vi "PH_PILS.Action _Cerpass.vi"(0 "i ref in":refnum<vi>, 2 "Service Name":string="N/A", 5 "error in":errorcluster) -> (14 "i ref out":refnum<vi>, 19 "error out":errorcluster)   [LabVIEW 2014, in "PH_PILS.lvlib"]
doc: "This VI sets the Cerpass GUI element."
uses:
  PH_PILS.lvlib
  PH_PILS.Operation Mode.ctl
  PH_Basics/PH_Common/PH_Common.lvlib
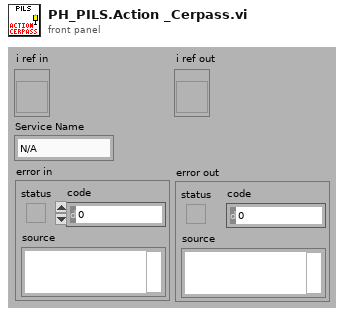
[diagram p1: front panel]
types:
  T1 = typedef "PH_PILS.lvlib/PH_PILS.Operation Mode.ctl" = enum16{"unknown", "Service", "Labor", "Search", "Shot"}
  T2 = typedef "PH_PILS.lvlib/PH_PILS.i attribute.ctl" = cluster{"Boolean":cluster{"GUI Ref":refnum<vi>, "Status":i32}[], "GUI Refs Exp. Shutters":cluster{"1":refnum<vi>, "2":refnum<vi>, "3":refnum<vi>, "4":refnum<vi>}, "Tristate2Run GUI Refs":refnum<vi>[], "EO-Likes":cluster{"GUI Ref":refnum<vi>, "Status":i32}[], "Operation Mode":cluster{"Operation Mode":T1, "GUI":cluster{"Ref State":refnum<vi>, "Ref":refnum<vi>}, "Servicemode":cluster{"Tagname":string, "Status":i32}, "Labormode":cluster{"Tagname":string, "Status":i32}, "Searchmode":cluster{"Tagname":string, "Status":i32}, "Shotmode":cluster{"Tagname":string, "Status":i32}}, "Submode":cluster{"Submode":T3, "GUI":cluster{"Ref State":refnum<vi>, "Ref":refnum<vi>}, "Submode":cluster{"Tagname":string, "Status":i32}}, "Experiment":cluster{"Experiment":enum16{"unknown", "intern", "4 (Z6)", "3", "2", "1"}, "GUI":cluster{"Ref State":refnum<vi>, "Ref":refnum<vi>}, "intern":cluster{"Tagname":string, "Status":i32}, "Exp 4":cluster{"Tagname":string, "Status":i32}, "Exp 3":cluster{"Tagname":string, "Status":i32}, "Exp 2":cluster{"Tagname":string, "Status":i32}, "Exp 1":cluster{"Tagname":string, "Status":i32}}, "TristateNormal":cluster{"GUI Ref":refnum<vi>, "Status":i32}[], "Door Tags":cluster{"GUI Ref":refnum<vi>, "Status":i32}[], "GUIlessTags":cluster{"Name":string, "Status":i32}[], "Beamline GUI Refs":refnum<vi>[], "Special Boolean":cluster{"GUI Ref":refnum<vi>, "Status":i32}[], "Laserpower":cluster{"GUI Ref":refnum<vi>, "Status":i32}[], "Shutter":cluster{"GUI Ref":refnum<vi>, "Status":i32}[], "Tristate EO Like":cluster{"GUI Ref":refnum<vi>, "Status":i32}[], "PP":cluster{"GUI Ref":refnum<vi>, "Status":i32, "Head Ref":refnum<vi>, "Slider Ref":refnum<vi>}[], "Switch Knobs":cluster{"GUI Ref":refnum<vi>, "Status":i32}[], "Latch Knob GUI Refs":refnum<vi>[], "FailureCounter":i32, "Enabled Status":cluster{"Laser":i32, "PreAmp":i32, "MainAmp":i32}, "Mercury":refnum<vi>, "Instance Rods":string, "Logfile":path, "Beckhoff-Instance Internal":string, "Beckhoff-Instance External":string, "Enabling Rights":cluster{"Name":string, "Password":string, "PA?":bool, "MA?":bool, "Exp?":bool}[]}
  T3 = typedef "PH_PILS.lvlib/PH_PILS.Submode.ctl" = enum16{"unknown", "HV-Normal", "HV-Test"}
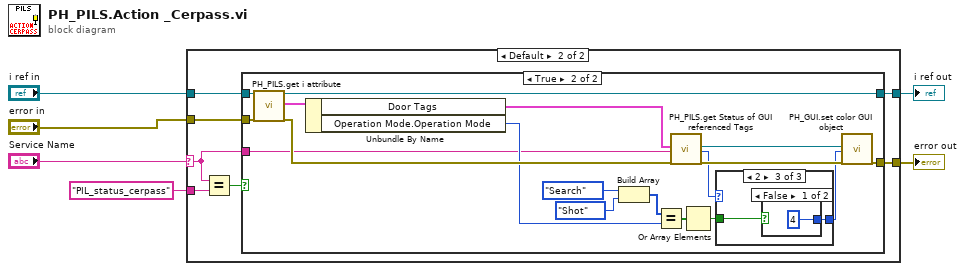
[diagram p0: block diagram]
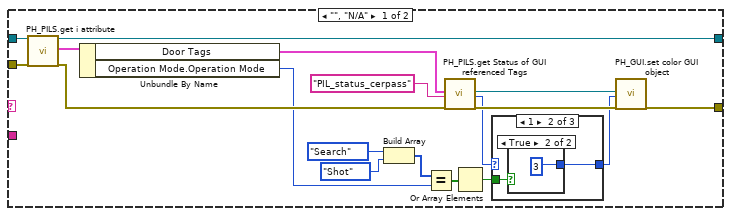
[diagram p2: hidden frame]
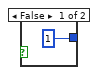
[diagram p4: hidden frame]
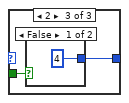
[diagram p5: hidden frame]
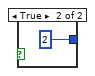
[diagram p6: hidden frame]
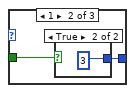
[diagram p9: hidden frame]
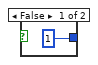
[diagram p10: hidden frame]
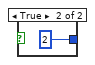
[diagram p11: hidden frame]
diagram:
  n1 = case shown="Default" "Service Name" {
    selector: "Service Name" -> [_ w36]
    tunnel: "error in" -> [w24 w40]
    tunnel: "i ref in" -> [w23 w39]
    tunnel: [w22 w38] -> w4
    tunnel: [w16 w37] -> w3
    tunnel: "PIL_status_cerpass" -> [_ w35]
    frame "", "N/A" {
      n2 = call "PH_PILS.get i attribute.vi"("i ref in"=w23, "error in (no error)"=w24) -> ("i ref out"=w22:refnum<vi>, "i attribute"=w21:T2, "error out"=w20:errorcluster)  [unwired: 15 in]
      n3 = Unbundle By Name(w21) -> ("Door Tags"=w18:cluster{"GUI Ref":refnum<vi>, "Status":i32}[], "Operation Mode.Operation Mode"=w9:T1)
      n4 = Build Array(PH_PILS.Operation_Mode."Search" ("Operation Mode.Operation Mode"), PH_PILS.Operation_Mode."Shot" ("Operation Mode.Operation Mode")) -> (w10:T1[])
      n5 = Equal?(x=w10, y=w9) -> (x = y?=w8:bool[])
      n6 = call "PH_PILS.get Status of GUI referenced Tags.vi"("Tags"=w18, "Tagname"="PIL_status_cerpass", "error in"=w20) -> ("GUI Ref"=w15:refnum<vi>, "Status"=w14:i32, "error out"=w17:errorcluster)  [unwired: 13 in, 1 out]
      n7 = Or Array Elements(Boolean array=w8) -> (logical OR=w7:bool)
      n8 = case shown="1" w14 {
        selector: w14 -> [w25 _ _]
        tunnel: [w25 w27 w31] -> w13
        tunnel: w7 -> [_ w26 w30]
        frame 0, Default {
        }
        frame 1 {
          n9 = case shown="True" w26 {
            tunnel: [1 3] -> w27
            frame False {
            }
            frame True {
            }
          }
        }
        frame 2 {
          n10 = case shown="False" w30 {
            tunnel: [4 2] -> w31
            frame False {
            }
            frame True {
            }
          }
        }
      }
      n11 = call "PH_GUI.set color GUI object.vi"("GUI object Ref"=w15, "State"=w13, "error in (no error)"=w17) -> ("error out"=w16:errorcluster)  [unwired: 16 in]
    }
    frame Default {
      n12 = Equal?(x=w36, y=w35) -> (x = y?=w34:bool)
      n13 = case shown="True" w34 {
        tunnel: w40 -> [w41 w60]
        tunnel: w39 -> [w42 w59]
        tunnel: [w42 w58] -> w38
        tunnel: [w41 w53] -> w37
        tunnel: w36 -> [_ w43]
        frame False {
        }
        frame True {
          n14 = call "PH_PILS.get i attribute.vi"("i ref in"=w59, "error in (no error)"=w60) -> ("i ref out"=w58:refnum<vi>, "i attribute"=w57:T2, "error out"=w56:errorcluster)  [unwired: 15 in]
          n15 = Unbundle By Name(w57) -> ("Door Tags"=w55:cluster{"GUI Ref":refnum<vi>, "Status":i32}[], "Operation Mode.Operation Mode"=w46:T1)
          n16 = Build Array(PH_PILS.Operation_Mode."Search" ("Operation Mode.Operation Mode"), PH_PILS.Operation_Mode."Shot" ("Operation Mode.Operation Mode")) -> (w47:T1[])
          n17 = Equal?(x=w47, y=w46) -> (x = y?=w45:bool[])
          n18 = call "PH_PILS.get Status of GUI referenced Tags.vi"("Tags"=w55, "Tagname"=w43, "error in"=w56) -> ("GUI Ref"=w52:refnum<vi>, "Status"=w51:i32, "error out"=w54:errorcluster)  [unwired: 13 in, 1 out]
          n19 = Or Array Elements(Boolean array=w45) -> (logical OR=w44:bool)
          n20 = case shown="2" w51 {
            selector: w51 -> [w61 _ _]
            tunnel: [w61 w63 w67] -> w50
            tunnel: w44 -> [_ w62 w66]
            frame 0, Default {
            }
            frame 1 {
              n21 = case shown="True" w62 {
                tunnel: [1 3] -> w63
                frame False {
                }
                frame True {
                }
              }
            }
            frame 2 {
              n22 = case shown="False" w66 {
                tunnel: [4 2] -> w67
                frame False {
                }
                frame True {
                }
              }
            }
          }
          n23 = call "PH_GUI.set color GUI object.vi"("GUI object Ref"=w52, "State"=w50, "error in (no error)"=w54) -> ("error out"=w53:errorcluster)  [unwired: 16 in]
        }
      }
    }
  }
  "error out" <- w3
  "i ref out" <- w4
